vi "Receive Message.vi"(6 "priority":i32, 10 "LoggingActor in":refnum<class "LoggingActor.lvclass">, 11 "Message in":refnum<class "Message.lvclass">) -> (0 "error out":errorcluster, 2 "Actor out":refnum<class "Actor.lvclass">)   [LabVIEW 2022 SP3, in "LoggingActor.lvlib" / "LoggingActor.lvclass"]
doc: "This VI should be overriden ONLY if you are creating a proxy actor for remote transmission. If you are, override this VI to transmit the received message to a new destination, maintaining the given priority."
uses:
  LoggingActor.lvclass
  LoggingActor.lvclass/LoggingActor.ctl
  <vilib>/ActorFramework/Actor/Actor.lvclass
  Logger/Source/Logger/Logger.lvclass
  <vilib>/ActorFramework/Message/Message.lvclass
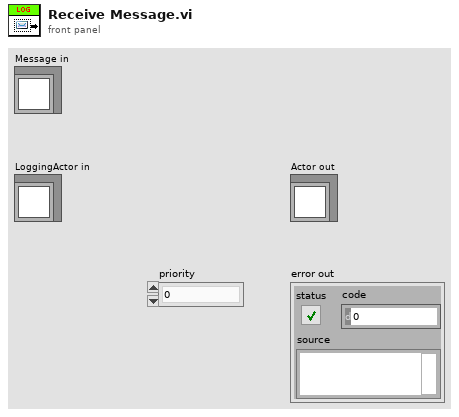
[diagram p1: front panel]
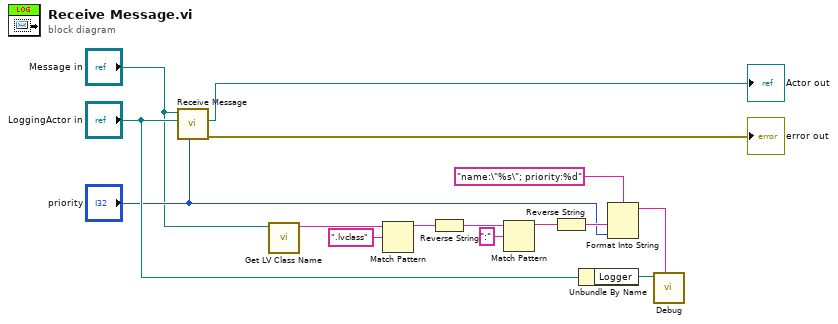
[diagram p0: block diagram]
diagram:
  n1 = call-parent "Receive Message.vi"("priority"="priority", "Actor in"="LoggingActor in", "Message in"="Message in") -> ("error out"=→"error out":errorcluster, "Actor out"=→"Actor out":refnum<class "Actor.lvclass">)  [unwired: 7 in]
  n2 = call <vilib>:"Get LV Class Name.vi"("object"="Message in") -> ("class name"=w9:string)  [unwired: 9 in, 1 out]
  n3 = Match Pattern(string=w9, regular expression=".lvclass") -> (before substring=w8:string)  [unwired: 1 in, 3 out]
  n4 = Reverse String(1:w8) -> (0:w6:string)
  n5 = Match Pattern(string=w6, regular expression=":") -> (before substring=w5:string)  [unwired: 1 in, 3 out]
  n6 = Reverse String(1:w5) -> (0:w3:string)
  n7 = Unbundle By Name("LoggingActor in") -> ("Logger"=w12:refnum<class "Logger.lvclass">)
  n8 = Format Into String(format string="name:\"%s\"; priority:%d", w3, "priority") -> (resulting string=w11:string)  [unwired: 2 in, 1 out]
  n9 = call-dynamic "Debug.vi"("Message"=w11, "Logger in"=w12) -> ()  [unwired: 6 in, 2 out]
